vi "Init Data Handling.vi"(4 "Channels per Group":cluster{"Channels":string[]}[](array[cluster]), 6 "Groups":string[](array[string]), 8 "error in (no error)":errorcluster, 9 "Channels":string[](array[string]), 10 "Buffer Size":i32, 11 "LocalGraphBuffer in":refnum<class "LocalGraphBuffer.lvclass">) -> (0 "error out":errorcluster, 3 "LocalGraphBuffer out":refnum<class "LocalGraphBuffer.lvclass">)   [LabVIEW 2020, in "VolatusGUIElements.lvlib" / "LocalGraphBuffer.lvclass"]
uses:
  LocalGraphBuffer.lvclass
  LocalGraphBuffer.lvclass/LocalGraphBuffer.ctl
  Plot.ctl
  <vilib>/Utility/miscctls.llb/LVMapReplaceAction.ctl
  lv-vecto/Vecto/Subscribed Data.ctl
  lv-vecto/Vecto/Vecto.lvlib
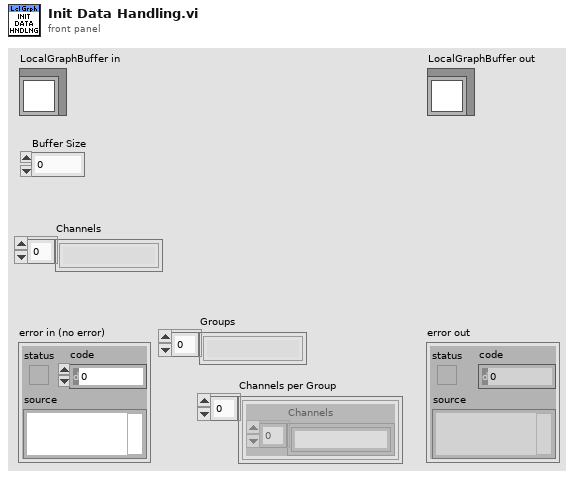
[diagram p1: front panel]
types:
  T1 = typedef "Vecto.lvlib/Subscribed Data.ctl" = cluster{"Group":string, "Timestamp":dbl, "Data":dbl[]}
  T2 = typedef "VolatusGUIElements.lvlib/LocalGraphBuffer.lvclass/Plot.ctl" = cluster{"Data Q":refnum<queue>, "Time Q":refnum<queue>, "Group":string}
  T3 = typedef "VolatusGUIElements.lvlib/LocalGraphBuffer.lvclass/Group Sub.ctl" = cluster{"Plot Indices":i32[]}
  T4 = typedef "LVMapReplaceAction.ctl" = enum32{"Modify Entry only if found", "Add or Modify Entry", "Delete Entry"}
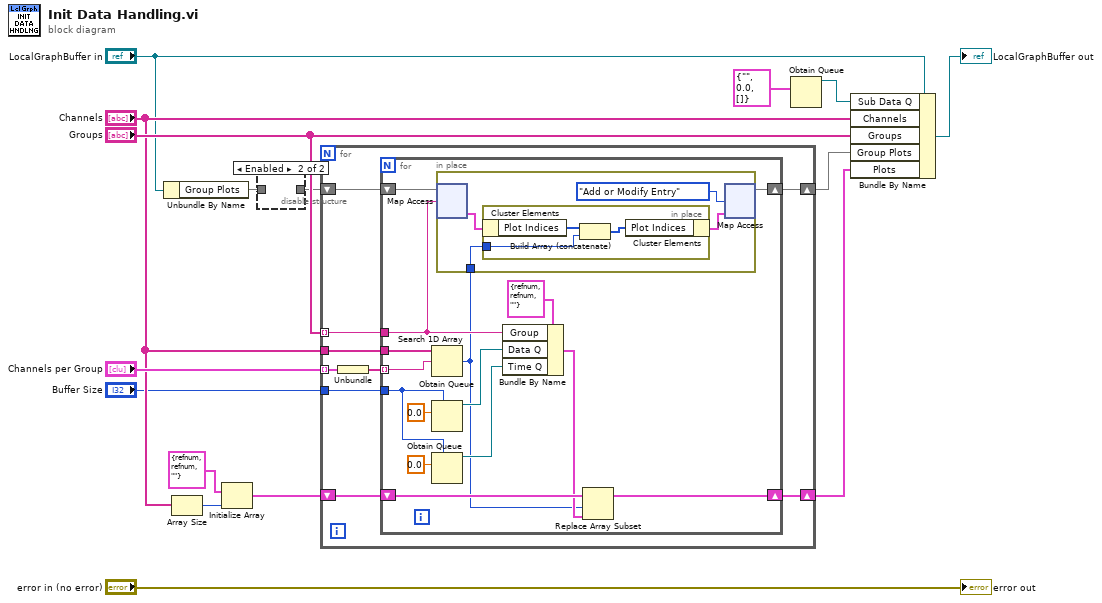
[diagram p0: block diagram]
diagram:
  n1 = Unbundle By Name("LocalGraphBuffer in") -> ("Group Plots"=w5:map{string, T3})
  n2 = Array Size(array="Channels") -> (size(s)=w12:i32)
  n3 = Initialize Array(T2 {"Data Q"=refnum, "Time Q"=refnum, "Group"=""} ("Plot"), w12) -> (w10:T2[])
  n4 = disable-structure shown="Enabled" {
    disable-tunnel: [w17 _] -> w6
    disable-tunnel: w5 -> [w17 _]
    frame Disabled {
    }
    frame Enabled {
    }
  }
  n5 = for {
    tunnel: "Groups" -> [w22] mode=indexing
    tunnel: "Channels per Group" -> [w26] mode=indexing
    shift-right: [w21] -> w8
    shift-left: w10 -> [w23]
    tunnel: "Channels" -> [w25]
    shift-right: [w19] -> w4
    shift-left: w6 -> [w20]
    tunnel: "Buffer Size" -> [w18]
    n6 = Unbundle(w26) -> ("Channels"=w24:string[])
    n7 = for {
      tunnel: w25 -> [w41]
      tunnel: w24 -> [w40] mode=indexing
      shift-right: [w32] -> w21
      shift-left: w23 -> [w34]
      tunnel: w22 -> [w30]
      shift-right: [w29] -> w19
      shift-left: w20 -> [w31]
      tunnel: w18 -> [w27]
      n8 = Search 1D Array(1D array=w41, element=w40) -> (index of element=w28:i32)  [unwired: 1 in]
      n9 = Obtain Queue(max queue size (-1, unlimited)=w27, element data type=0.0) -> (queue out=w37:refnum<queue>)  [unwired: 3 in, 2 out]
      n10 = Obtain Queue(max queue size (-1, unlimited)=w27, element data type=0.0) -> (queue out=w35:refnum<queue>)  [unwired: 3 in, 2 out]
      n11 = in-place {
        in-place-border: w28 -> [w42]
        n12 = in-place-map #1(w31, w30) -> (w44:T3)  [unwired: 1 in, 1 out]
        n13 = in-place {
          in-place-border: w42 -> [w46]
          n14 = in-place-cluster #2(w44) -> ("Plot Indices"=w48:i32[])
          n15 = Build Array (concatenate)(w48, w46) -> (w47:i32[])
          n16 = in-place-cluster #2("Plot Indices"=w47) -> (w43:T3)
        }
        n17 = in-place-map #1(w43, LVMapReplaceAction."Add or Modify Entry" ("action")) -> (w29:map{string, T3})  [unwired: 2 out]
      }
      n18 = Bundle By Name(cluster=T2 {"Data Q"=refnum, "Time Q"=refnum, "Group"=""} ("Plot"), "Group"=w30, "Data Q"=w37, "Time Q"=w35) -> (w33:T2)
      n19 = Replace Array Subset(array=w34, new element=w33, index=w28) -> (w32:T2[])
    }
  }
  n20 = Obtain Queue(element data type=T1 {"Group"="", "Timestamp"=0.0, "Data"=[]} ("Subscribed Data")) -> (queue out=w1:refnum<queue>)  [unwired: 4 in, 2 out]
  n21 = Bundle By Name(cluster="LocalGraphBuffer in", "Sub Data Q"=w1, "Channels"="Channels", "Groups"="Groups", "Group Plots"=w4, "Plots"=w8) -> (→"LocalGraphBuffer out":refnum<class "LocalGraphBuffer.lvclass">)
  "error out" <- "error in (no error)"
